vi "write to file practice.vi"() -> ()   [LabVIEW 2014]
panel:
  in  "stop":bool
  in  "access (0:read/write)":enum16{"read/write", "read-only", "write-only"}(ring)
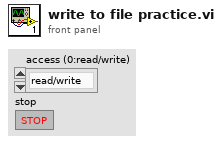
[diagram p1: front panel]
types:
  T1 = enum16{"open", "replace", "create", "open or create", "replace or create", "replace or create with confirmation"}
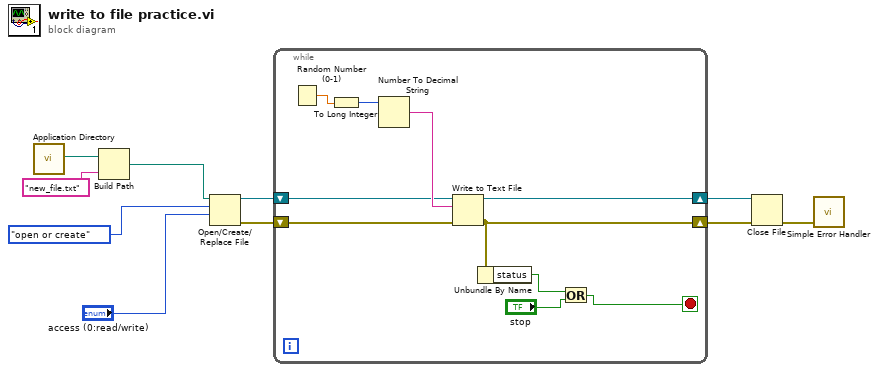
[diagram p0: block diagram]
diagram:
  n1 = call <vilib>:"Application Directory.vi"() -> ("Application Directory"=w3:path)
  n2 = Build Path(base path=w3, name or relative path="new_file.txt") -> (appended path=w1:path)
  n3 = Open/Create/Replace File(file path (use dialog)=w1, operation (0:open)=T1."open or create", access (0:read/write)="access (0:read/write)") -> (refnum out=w7:refnum<file>, error out=w8:errorcluster)  [unwired: 3 in, 1 out]
  n4 = while {
    shift-right: [w16] -> w5
    shift-left: w8 -> [w20]
    shift-right: [w17] -> w6
    shift-left: w7 -> [w18]
    stop <- w13 stop-if-true
    n5 = Random Number (0-1)() -> (number: 0 to 1=w11:dbl)
    n6 = To Long Integer(number=w11) -> (32bit integer=w12:i32)
    n7 = Number To Decimal String(number=w12) -> (decimal integer string=w19:string)  [unwired: 1 in]
    n8 = Write to Text File(file (use dialog)=w18, text=w19, error in=w20) -> (refnum out=w17:refnum<file>, error out=w16:errorcluster)  [unwired: 1 in, 1 out]
    n9 = Unbundle By Name(w16) -> ("status"=w15:bool)
    n10 = Or(x=w15, y="stop") -> (x .or. y?=w13:bool)
  }
  n11 = Close File(refnum=w6, error in=w5) -> (error out=w4:errorcluster)  [unwired: 1 out]
  n12 = call <vilib>:"Simple Error Handler.vi"("error in (no error)"=w4) -> ()  [unwired: 4 in, 5 out]
